vi "does_plane_hit.vi"(8 "error in (no error)":errorcluster, 10 "depth":dbl[unit], 11 "RoiGeneric.lvclass in":refnum<class "RoiGeneric.lvclass">) -> (0 "error out":errorcluster, 2 "is hit?":bool, 3 "RoiGeneric.lvclass out":refnum<class "RoiGeneric.lvclass">)   [LabVIEW 2010, in "RoiGeneric.lvclass"]
uses:
  RoiGeneric.lvclass
  common/classes/Box/Box/Box.lvclass
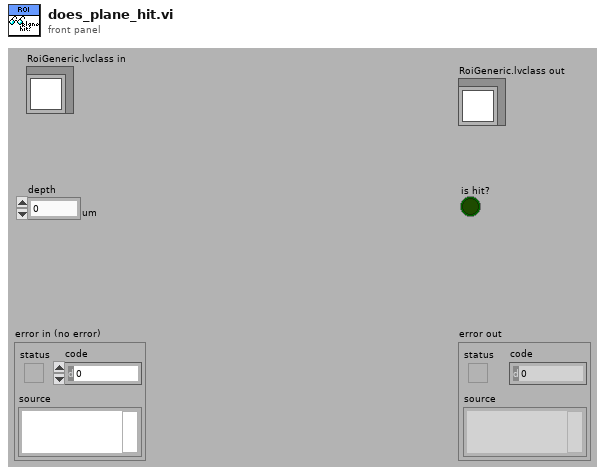
[diagram p1: front panel]
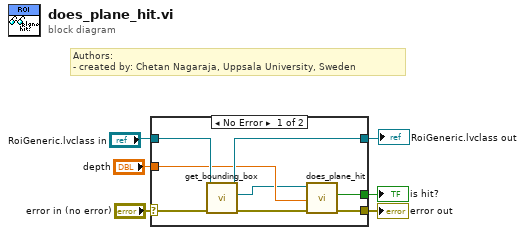
[diagram p0: block diagram]
diagram:
  # "Authors: \n- created by: Chetan Nagaraja, Uppsala University, Sweden"
  n1 = case shown="No Error" "error in (no error)" {
    selector: "error in (no error)" -> [w14 w16]
    tunnel: [w10 w16] -> w5
    tunnel: [w12 w15] -> w2
    tunnel: "RoiGeneric.lvclass in" -> [w13 w15]
    tunnel: "depth" -> [w9 _]
    tunnel: [w8 _] -> w3
    frame No Error {
      n2 = call-dynamic "get_bounding_box.vi"("error in (no error)"=w14, "RoiGeneric in"=w13) -> ("error out"=w11:errorcluster, "Box.lvclass"=w7:refnum<class "Box.lvclass">, "RoiGeneric out"=w12:refnum<class "RoiGeneric.lvclass">)  [unwired: 7 in]
      n3 = call "does_plane_hit.vi"("error in (no error)"=w11, "depth"=w9, "Box in"=w7) -> ("error out"=w10:errorcluster, "is inside?"=w8:bool)  [unwired: 6 in, 1 out]
    }
    frame Error {
    }
  }
  "error out" <- w5
  "is hit?" <- w3
  "RoiGeneric.lvclass out" <- w2
